vi "window_coeff.vi"(6 "window":T1(ring), 9 "tone frequency [Hz]":dbl=1000.0 format="%.2f", 10 "Numeric in":i32, 11 "df":dbl) -> (1 "Array 2":cdb[](array[numeric]), 2 "Array":cdb[](array[numeric]), 3 "Numeric out":i32)   [LabVIEW 2021]
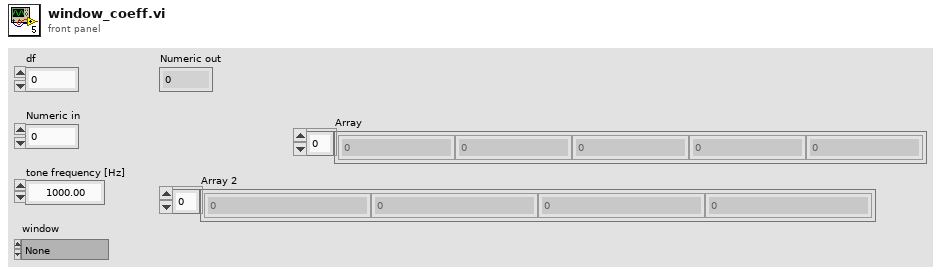
[diagram p1: front panel]
types:
  T1 = enum16{"None ", "Hanning", "Hamming", "Blackman-Harris", "Exact Blackman", "Blackman", "Flat Top", "4 Term B-Harris ", "7 Term B-Harris", "Low Sidelobe"}
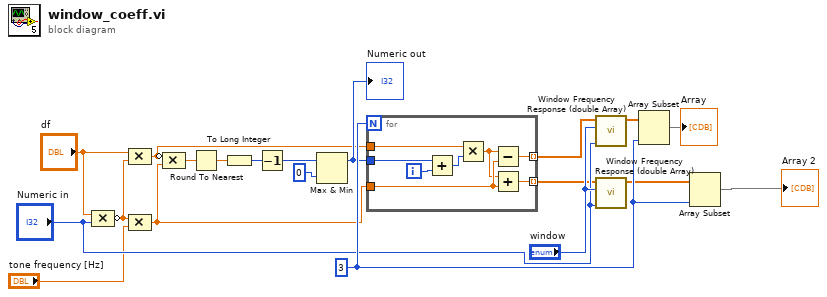
[diagram p0: block diagram]
diagram:
  w20 = 3
  n1 = Compound Arithmetic op=MULTIPLY("df", "Numeric in") -> (invert w2:dbl)
  n2 = Compound Arithmetic op=MULTIPLY("df", w2) -> (w6:dbl)
  n3 = Compound Arithmetic op=MULTIPLY(w2, "tone frequency [Hz]") -> (w16:dbl)
  n4 = Compound Arithmetic op=MULTIPLY(invert w6, w16) -> (w5:dbl)
  n5 = Round To Nearest(number=w5) -> (nearest integer value=w4:dbl)
  n6 = To Long Integer(number=w4) -> (32bit integer=w3:i32)
  n7 = Decrement(x=w3) -> (x-1=w7:i32)
  n8 = Max & Min(x=w7, y=0) -> (max(x,y)=w9:i32)  [unwired: 1 out]
  "Numeric out" <- w9
  n9 = for {
    N: w20 -> [_]
    tunnel: w6 -> [w25]
    tunnel: w16 -> [w28]
    tunnel: [w27] -> w15 mode=indexing
    tunnel: [w26] -> w14 mode=indexing
    tunnel: w9 -> [w24]
    i -> [w22]
    n10 = Add(x=w24, y=w22) -> (x+y=w23:i32)
    n11 = Multiply(x=w25, y=w23) -> (x*y=w21:dbl)
    n12 = Subtract(x=w21, y=w28) -> (x-y=w27:dbl)
    n13 = Add(x=w21, y=w28) -> (x+y=w26:dbl)
  }
  n14 = call "Window Frequency Response (double Array).vi"("N (window length)"="Numeric in", "window"="window", "f(normalized)"=w15) -> ("H(f)"=w12:cdb[])  [unwired: 8 in]
  n15 = call "Window Frequency Response (double Array).vi"("N (window length)"="Numeric in", "window"="window", "f(normalized)"=w14) -> ("H(f)"=w13:cdb[])  [unwired: 8 in]
  n16 = Array Subset(array=w12, length=w20) -> (→"Array":cdb[])  [unwired: 1 in]
  n17 = Array Subset(array=w13, length=w20) -> (→"Array 2":cdb[])  [unwired: 1 in]
